vi "430_GPIB_Command.vi"(0 "GPIB (In)":cluster{"GPIB address":i16, "GPIB bus":i16}={"GPIB address"=15, "GPIB bus"=0}, 1 "Input command":string, 2 "error in":T1) -> (3 "GPIB (Out)":cluster{"GPIB address":i16, "GPIB bus":i16}={"GPIB address"=15, "GPIB bus"=0}, 4 "Bytes sent":i32, 5 "Return string":string, 6 "error out":T1)   [LabVIEW 2017]
doc: "Implements a GPIB command given the GPIB bus information and the input command string. The *OPC? query is sent after each command for handshaking purposes.\n\nMultiple serial polls are performed as required after sending the *OPC? command in order to determine when bit 4 (GPIB MESSAGE AVAILABLE) is set indicating the return data is available. Instruments must support the IEEE 488.2 spec for the serial poll byte for this VI to work correctly.\n\nThe *OPC? timeout setting (internal to VI) limits the amount of time the VI will wait for bit 4 to be set by the instrument."
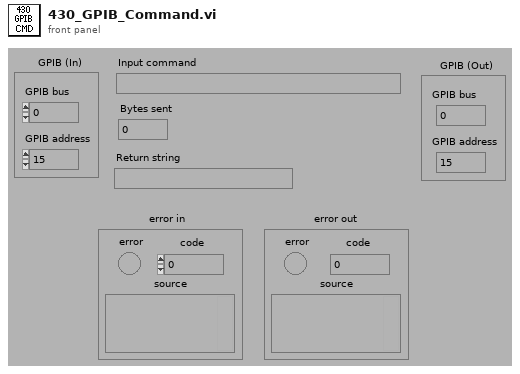
[diagram p1: front panel]
types:
  T1 = cluster{"error":bool, "code":i32, "source":string}
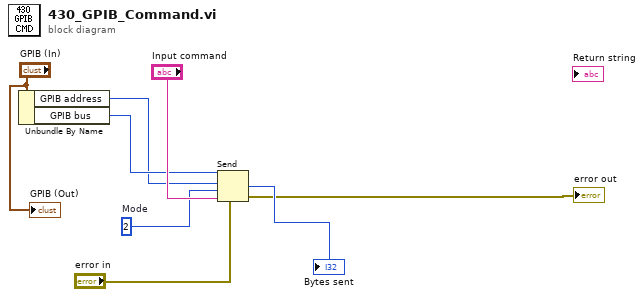
[diagram p0: block diagram]
diagram:
  w5 = u8 2  # Mode
  n1 = Unbundle By Name("GPIB (In)") -> ("GPIB address"=w2:i16, "GPIB bus"=w3:i16)
  n2 = Send(0:w3, 2:w2, 3:w5, 4:"error in", 5:"Input command") -> (7:→"Bytes sent":i32, 8:→"error out":errorcluster)  [unwired: 1 out]
  "GPIB (Out)" <- "GPIB (In)"
